vi "PH_BeamlineController.set current Value of Source Elements in Case of none Targets.vi"(0 "VI in":refnum<vi>, 5 "error in (no error)":errorcluster) -> (14 "VI out":refnum<vi>, 19 "error out":errorcluster)   [LabVIEW 2014, in "PH_BeamlineController.lvlib"]
uses:
  PH_BeamlineController.lvlib
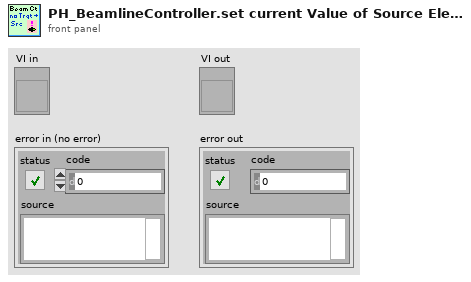
[diagram p1: front panel]
types:
  T1 = typedef "PH_BeamlineController.lvlib/PH_BeamlineController.i attribute.ctl" = cluster{"Vacuum Exp LB":cluster{"Channel":string, "Limit [mbar]":dbl, "Pressure [mbar]":dbl, "GUI Ref":refnum<vi>}, "Sources":T2[], "PA DP Targets":T4[], "Path":cluster{"Source":T3, "PA DP Target":T5, "Target":T6}, "Targets":cluster{"Name":T6, "GUI Ref":refnum<vi>, "Current State":bool, "Wanted State":bool, "Enabled":bool}[], "Status Tags":cluster{"Name":string, "Status":T7}[], "special GUI Refs":T8}
  T2 = typedef "PH_BeamlineController.lvlib/PH_BeamlineController.Source Attributes.ctl" = cluster{"Name":T3, "GUI Ref":refnum<vi>, "Current State":bool, "Wanted State":bool}
  T3 = typedef "PH_BeamlineController.lvlib/PH_BeamlineController.Sources.ctl" = enum16{"None", "YLF", "fs-Frontend", "ns-Frontend", "YLF and ns-Frontend", "fs- and ns-Frontend"}
  T4 = typedef "PH_BeamlineController.lvlib/PH_BeamlineController.PA DP Target Attributes.ctl" = cluster{"Name":T5, "GUI Ref":refnum<vi>, "Current State":bool, "Wanted State":bool, "Enabled":bool}
  T5 = typedef "PH_BeamlineController.lvlib/PH_BeamlineController.PA DP Targets.ctl" = enum16{"None", "Dump PA Delayed Beam", "Dump PA Undelayed Beam", "Dumps PA Delayed and Undelayed Beam"}
  T6 = typedef "PH_BeamlineController.lvlib/PH_BeamlineController.Targets.ctl" = enum16{"None", "PreAmp", "Dump Exp Laserlab", "Exp Laserlab", "Calorimeter", "Dump Exp Laserbay", "Exp Laserbay", "Dump Exp Z6", "Exp Z6"}
  T7 = typedef "PH_StatusHandler.lvlib/PH_StatusHandler.Status.ctl" = i16
  T8 = typedef "PH_BeamlineController.lvlib/PH_BeamlineController.special GUI Refs.ctl" = cluster{"PA-Backreflection-Meas":refnum<vi>, "fs_Synchrolock_Watch":refnum<vi>}
  T9 = cluster{"Name":T6, "GUI Ref":refnum<vi>, "Current State":bool, "Wanted State":bool, "Enabled":bool}[]
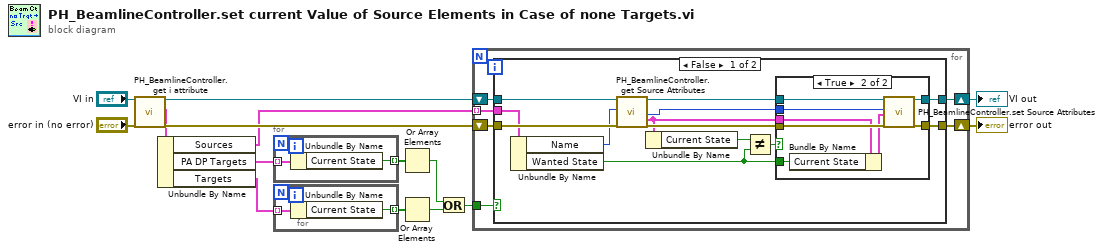
[diagram p0: block diagram]
diagram:
  n1 = call "PH_BeamlineController.get i attribute.vi"("i ref in"="VI in", "error in (no error)"="error in (no error)") -> ("i ref out"=w13:refnum<vi>, "i attribute"=w14:T1, "error out"=w15:errorcluster)  [unwired: 15 in]
  n2 = Unbundle By Name(w14) -> ("Sources"=w10:T2[], "PA DP Targets"=w7:T4[], "Targets"=w6:T9)
  n3 = for {
    tunnel: w7 -> [w17] mode=indexing
    tunnel: [w16] -> w5 mode=indexing
    n4 = Unbundle By Name(w17) -> ("Current State"=w16:bool)
  }
  n5 = for {
    tunnel: w6 -> [w19] mode=indexing
    tunnel: [w18] -> w4 mode=indexing
    n6 = Unbundle By Name(w19) -> ("Current State"=w18:bool)
  }
  n7 = Or Array Elements(Boolean array=w5) -> (logical OR=w3:bool)
  n8 = Or Array Elements(Boolean array=w4) -> (logical OR=w2:bool)
  n9 = Or(x=w3, y=w2) -> (x .or. y?=w1:bool)
  n10 = for {
    shift-right: [w25] -> w12
    shift-left: w15 -> [w22]
    shift-right: [w24] -> w11
    shift-left: w13 -> [w23]
    tunnel: w10 -> [w21] mode=indexing
    tunnel: w1 -> [w20]
    n11 = case shown="False" w20 {
      tunnel: [w37 w49] -> w25
      tunnel: [w35 w50] -> w24
      tunnel: w23 -> [w30 w50]
      tunnel: w22 -> [w29 w49]
      tunnel: w21 -> [w28 _]
      frame False {
        n12 = Unbundle By Name(w28) -> ("Name"=w27:T3, "Wanted State"=w26:bool)
        n13 = call "PH_BeamlineController.get Source Attributes.vi"("VI in"=w30, "Source"=w27, "error in (no error)"=w29) -> ("VI out"=w36:refnum<vi>, "Source Index"=w34:i32, "Source Attributes"=w33:T2, "error out"=w38:errorcluster)  [unwired: 13 in]
        n14 = Unbundle By Name(w33) -> ("Current State"=w32:bool)
        n15 = Not Equal?(x=w32, y=w26) -> (x != y?=w31:bool)
        n16 = case shown="True" w31 {
          tunnel: w38 -> [w39 w48]
          tunnel: [w39 w47] -> w37
          tunnel: w36 -> [w40 w46]
          tunnel: [w40 w45] -> w35
          tunnel: w34 -> [_ w44]
          tunnel: w33 -> [_ w42]
          tunnel: w26 -> [_ w41]
          frame False {
          }
          frame True {
            n17 = Bundle By Name(cluster=w42, "Current State"=w41) -> (w43:T2)
            n18 = call "PH_BeamlineController.set Source Attributes.vi"("VI in"=w46, "Source Index"=w44, "Changed Source Attributes"=w43, "error in (no error)"=w48) -> ("VI out"=w45:refnum<vi>, "error out"=w47:errorcluster)  [unwired: 14 in]
          }
        }
      }
      frame True {
      }
    }
  }
  "VI out" <- w11
  "error out" <- w12
